vi "GetAppRef.vi"() -> (0 "error out":errorcluster, 1 "App Refnum":refnum<vi>)   [LabVIEW 2012]
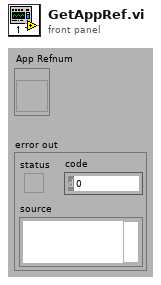
[diagram p1: front panel]
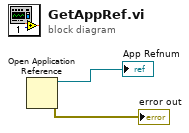
[diagram p0: block diagram]
diagram:
  n1 = Open Application Reference() -> (0:→"error out":errorcluster, 3:→"App Refnum":refnum<vi>)  [unwired: 1 in, 3 out]
